vi "Init Leds and Dut Selectors.vi"(7 "SWD Sel Lines (Clk, Dio, Rst)":tag, 8 "error in":errorcluster, 9 "RF Switch Sel Line":tag, 10 "Dut2 Pass Fail Lines":tag, 11 "Dut1 Pass Fail Lines":tag) -> (0 "error out":errorcluster, 1 "RF Switch Sel Task":refnum<k21>, 2 "Dut2 Leds Task":refnum<k21>, 3 "Dut1 Leds Task":refnum<k21>, 5 "SWD Sel Task":refnum<k21>)   [LabVIEW 2018]
uses:
  <vilib>/DAQmx/write.llb/DAQmx Write (Digital 1D Bool 1Chan 1Samp).vi
  <vilib>/DAQmx/write.llb/DAQmx Write (Digital Bool 1Line 1Point).vi
  <vilib>/DAQmx/create/channels.llb/DAQmx Create Channel (DO-Digital Output).vi
  <vilib>/DAQmx/miscellaneous.llb/DAQmx Fill In Error Info.vi
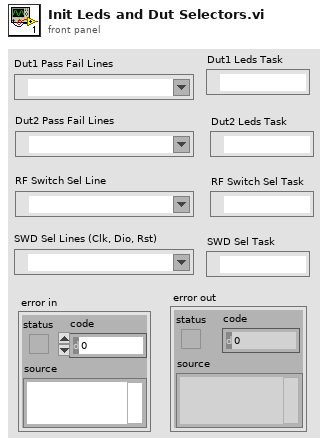
[diagram p1: front panel]
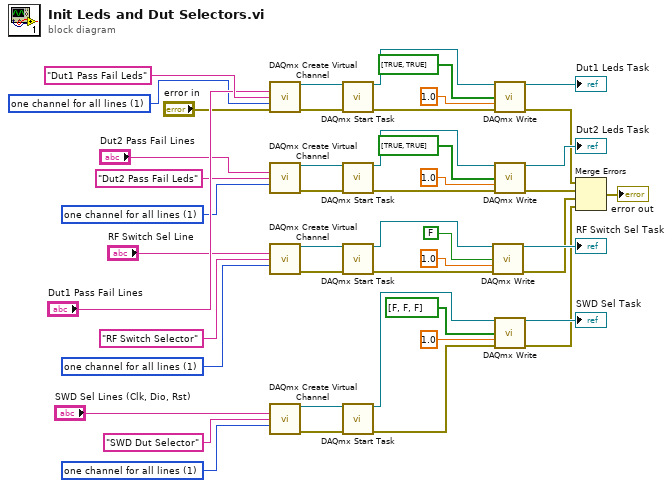
[diagram p0: block diagram]
diagram:
  w10 = 1 items=["one channel for each line", "one channel for all lines"] ("line grouping")
  w28 = 1 items=["one channel for each line", "one channel for all lines"] ("line grouping")
  w41 = 1 items=["one channel for each line", "one channel for all lines"] ("line grouping")
  w44 = 1 items=["one channel for each line", "one channel for all lines"] ("line grouping")
  n1 = call-poly <vilib>:"DAQmx Create Virtual Channel.vi"("lines"="Dut1 Pass Fail Lines", "name to assign"="Dut1 Pass Fail Leds" ("Dut1 Pass/Fail Leds"), "line grouping"=w44, "error in"="error in") -> ("task out"=w23:refnum<k21>, "error out"=w21:errorcluster)  [unwired: 10 in]
  n2 = call-poly <vilib>:"DAQmx Create Virtual Channel.vi"("lines"="Dut2 Pass Fail Lines", "name to assign"="Dut2 Pass Fail Leds" ("Dut1 Pass/Fail Leds"), "line grouping"=w41) -> ("task out"=w19:refnum<k21>, "error out"=w17:errorcluster)  [unwired: 11 in]
  n3 = call-poly <vilib>:"DAQmx Create Virtual Channel.vi"("lines"="RF Switch Sel Line", "name to assign"="RF Switch Selector" ("Dut1 Pass/Fail Leds"), "line grouping"=w28) -> ("task out"=w15:refnum<k21>, "error out"=w13:errorcluster)  [unwired: 11 in]
  n4 = call-poly <vilib>:"DAQmx Create Virtual Channel.vi"("lines"="SWD Sel Lines (Clk, Dio, Rst)", "name to assign"="SWD Dut Selector" ("Dut1 Pass/Fail Leds"), "line grouping"=w10) -> ("task out"=w6:refnum<k21>, "error out"=w4:errorcluster)  [unwired: 11 in]
  n5 = call <vilib>:"DAQmx Start Task.vi"("task/channels in"=w23, "error in"=w21) -> ("task out"=w22:refnum<k21>, "error out"=w20:errorcluster)  [unwired: 12 in]
  n6 = call <vilib>:"DAQmx Start Task.vi"("task/channels in"=w19, "error in"=w17) -> ("task out"=w18:refnum<k21>, "error out"=w16:errorcluster)  [unwired: 12 in]
  n7 = call <vilib>:"DAQmx Start Task.vi"("task/channels in"=w15, "error in"=w13) -> ("task out"=w14:refnum<k21>, "error out"=w12:errorcluster)  [unwired: 12 in]
  n8 = call <vilib>:"DAQmx Start Task.vi"("task/channels in"=w6, "error in"=w4) -> ("task out"=w5:refnum<k21>, "error out"=w3:errorcluster)  [unwired: 12 in]
  n9 = call-poly <vilib>:"DAQmx Write.vi"("task/channels in"=w14, "data"=FALSE, "timeout"=1.0, "error in"=w12) -> ("task out"=→"RF Switch Sel Task":refnum<k21>, "error out"=w25:errorcluster)  [unwired: 9 in, 1 out]
  n10 = call-poly <vilib>:"DAQmx Write.vi"("task/channels in"=w22, "data"=bool[] [TRUE, TRUE], "timeout"=1.0, "error in"=w20) -> ("task out"=→"Dut1 Leds Task":refnum<k21>, "error out"=w34:errorcluster)  [unwired: 9 in, 1 out]
  n11 = call-poly <vilib>:"DAQmx Write.vi"("task/channels in"=w18, "data"=bool[] [TRUE, TRUE], "timeout"=1.0, "error in"=w16) -> ("task out"=→"Dut2 Leds Task":refnum<k21>, "error out"=w33:errorcluster)  [unwired: 9 in, 1 out]
  n12 = call-poly <vilib>:"DAQmx Write.vi"("task/channels in"=w5, "data"=bool[] [FALSE, FALSE, FALSE], "timeout"=1.0, "error in"=w3) -> ("task out"=→"SWD Sel Task":refnum<k21>, "error out"=w1:errorcluster)  [unwired: 9 in, 1 out]
  n13 = Merge Errors(w34, w33, w25, w1) -> (→"error out":errorcluster)
